vi "Create Array (2D).vi"() -> ()   [LabVIEW 2019]
panel:
  out "Waveform Graph":dbl[][](graph)
  in  "My Numeric Array":dbl[][](array[numeric])=[[5.0, 10.0, 15.0, 20.0, 25.0], [3.0, 6.0, 9.0, 12.0, 15.0], [1.0, 2.0, 1.0, 2.0, 1.0]]
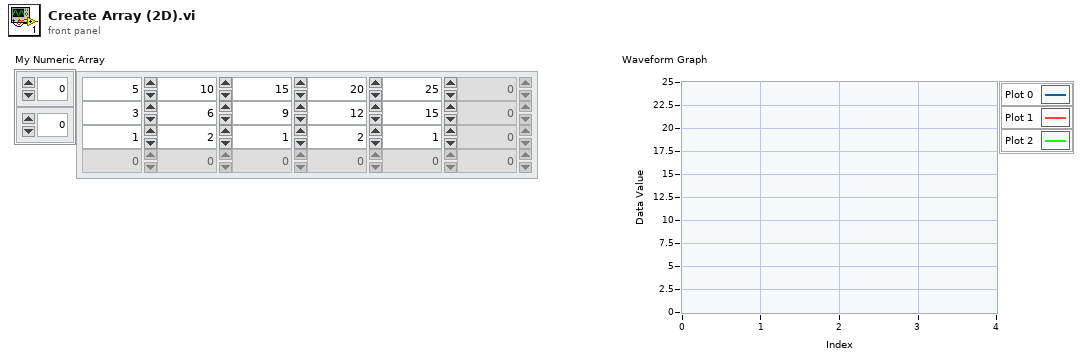
[diagram p1: front panel]
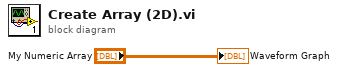
[diagram p0: block diagram]
diagram:
  "Waveform Graph" <- "My Numeric Array"
